vi "ReceiveNewMessage.vi"(8 "error in (no error)":errorcluster, 10 "Message Cluster":T1, 11 "Chat Room Model in":refnum<class "Chat Room Model.lvclass">) -> (0 "error out":errorcluster, 3 "Chat Room Model out":refnum<class "Chat Room Model.lvclass">)   [LabVIEW 2020, in "Chat Room Model.lvlib" / "Chat Room Model.lvclass"]
uses:
  Chat Room Model.lvclass
  Application Control/Message.ctl
  Chat Room Model.lvclass/Chat Room Model.ctl
  Chat Window UI Controller/Chat Window UI Controller Messages/Update Message Log Msg/Update Message Log Msg.lvclass/Update Message Log Msg.ctl
  <vilib>/ActorFramework/Message Enqueuer/Message Enqueuer.lvclass/Message Enqueuer.ctl
  <vilib>/ActorFramework/Message Enqueuer/Enqueue.vi
  Chat Window UI Controller/Chat Window UI Controller Messages/Update Message Log Msg/Update Message Log Msg.lvclass
  C:/Program Files (x86)/National Instruments/LabVIEW 2020/vi.lib/ActorFramework/Message/Message.lvclass
  <vilib>/ActorFramework/Message Priority Queue/Priority Enqueue.vi
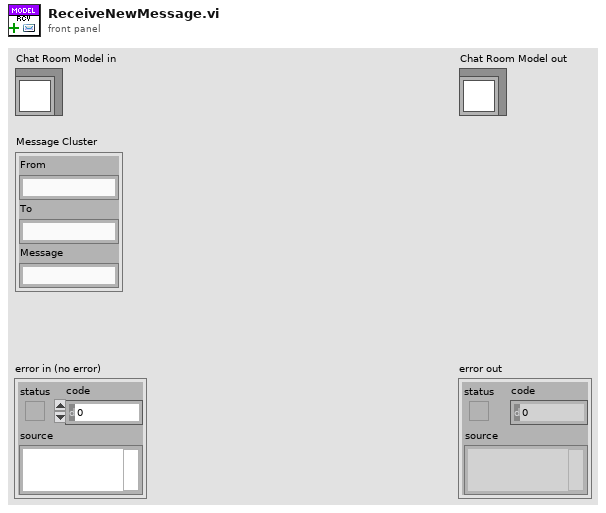
[diagram p1: front panel]
types:
  T1 = typedef "Message.ctl" = cluster{"From":string, "To":string, "Message":string}
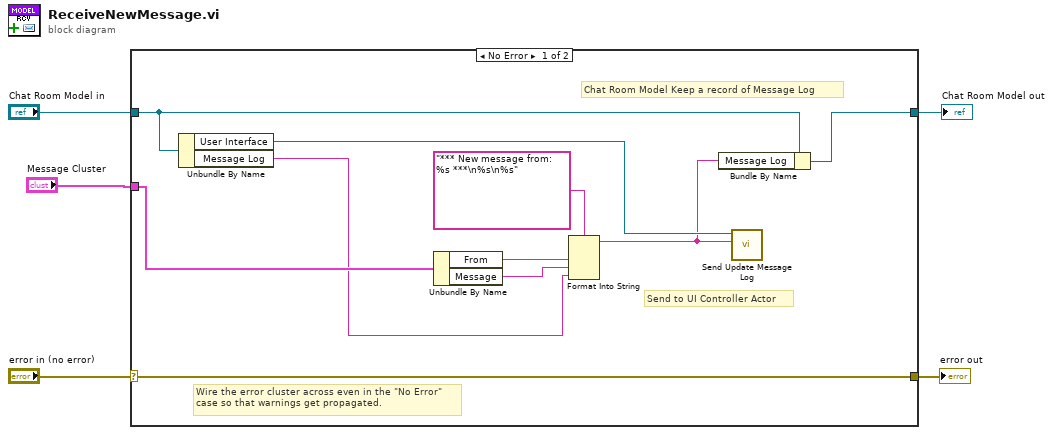
[diagram p0: block diagram]
diagram:
  n1 = case shown="No Error" "error in (no error)" {
    selector: "error in (no error)" -> [w15 w17]
    tunnel: [w15 w17] -> w4
    tunnel: [w9 w16] -> w2
    tunnel: "Chat Room Model in" -> [w11 w16]
    tunnel: "Message Cluster" -> [w12 _]
    frame No Error {
      # "Chat Room Model Keep a record of Message Log"
      # "Send to UI Controller Actor"
      # "Wire the error cluster across even in the \"No Error\"\ncase so that warnings get propagated."
      n2 = Unbundle By Name(w11) -> ("User Interface"=w14:refnum<class "Message Enqueuer.lvclass">, "Message Log"=w6:string)
      n3 = Unbundle By Name(w12) -> ("From"=w8:string, "Message"=w7:string)
      n4 = Format Into String(format string="*** New message from: %s ***\n%s\n%s", w8, w7, w6) -> (resulting string=w10:string)  [unwired: 2 in, 1 out]
      n5 = Bundle By Name(cluster=w11, "Message Log"=w10) -> (w9:refnum<class "Chat Room Model.lvclass">)
      n6 = call "Send Update Message Log.vi"("Newl Msg"=w10, "Message Enqueuer"=w14) -> ()  [unwired: 8 in, 2 out]
    }
    frame Error {
    }
  }
  "error out" <- w4
  "Chat Room Model out" <- w2
